vi "WVDIAL_2_Switch_v2.vi"() -> ()   [LabVIEW 2012]
uses:
  <vilib>/DAQmx/create/channels.llb/DAQmx Create Channel (CO-Pulse Generation-Ticks).vi
  <vilib>/DAQmx/configure/timing.llb/DAQmx Timing (Implicit).vi
  <resource>/objmgr/daqmx.rc
  <vilib>/DAQmx/create/channels.llb/DAQmx Create Channel (DO-Digital Output).vi
panel:
  in  "online":u32=2
  in  "offline":u32=2
  out "Error Out":errorcluster
  in  "stop 3":bool
  in  "Error In 3":errorcluster
  out "Error Out 3":errorcluster
  in  "Error In":errorcluster
  in  "Stop":bool
  in  "pulse counter":u32=140 min=4 max=9000 step=1
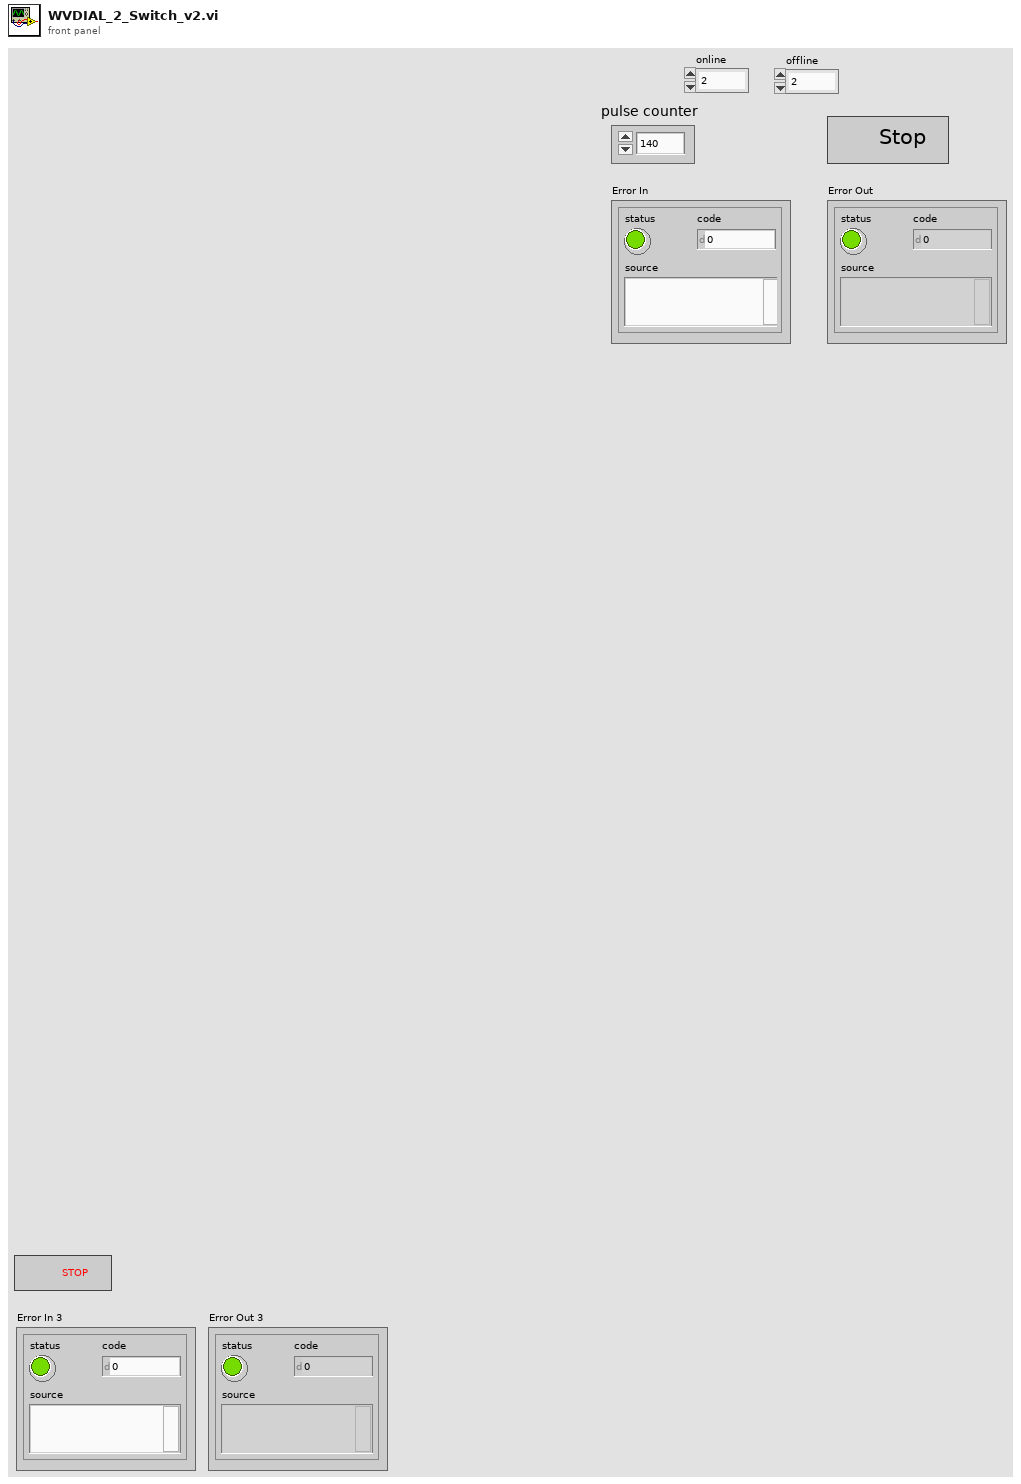
[diagram p1: front panel]
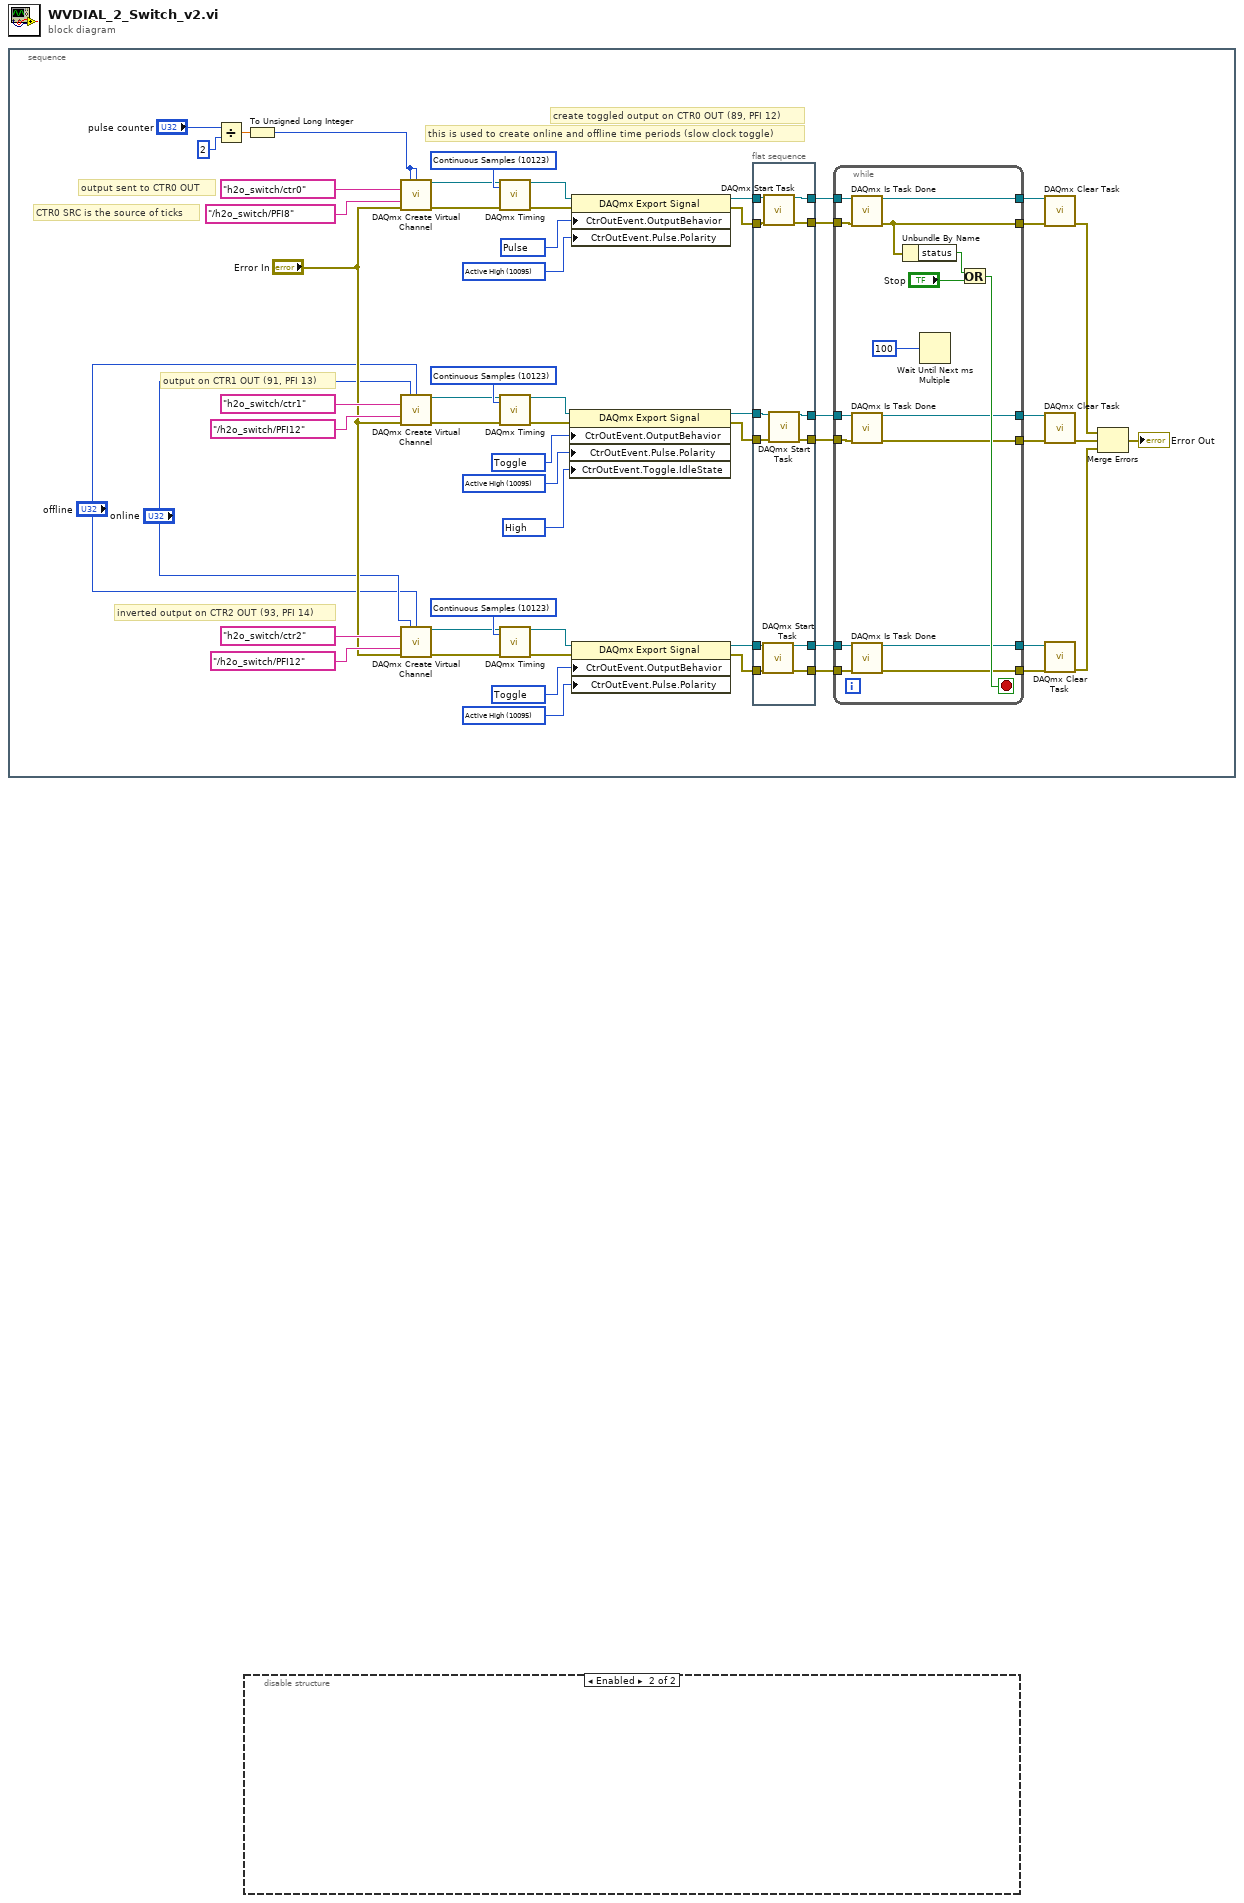
[diagram p0: block diagram]
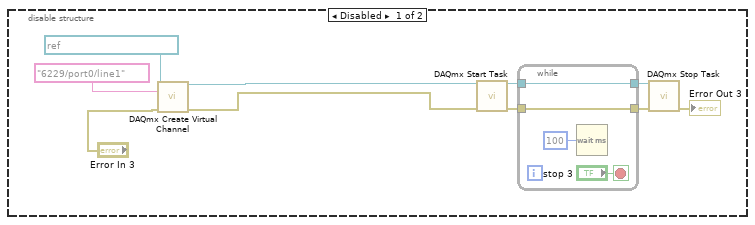
[diagram p2: hidden frame]
diagram:
  n1 = stacked-sequence {
    frame #0 {
      w11 = 10192 items=["High"=10192, "Low"=10214] ("CtrOutEvent.Toggle.IdleState")
      w21 = 10095 items=["Active High"=10095, "Active Low"=10096] ("CtrOutEvent.Pulse.Polarity")
      w27 = 10307 items=["Pulse"=10265, "Toggle"=10307] ("CtrOutEvent.OutputBehavior")
      w24 = 10123 items=["Finite Samples"=10178, "Continuous Samples"=10123, "Hardware Timed Single Point"=12522] ("sample mode")
      w38 = 10095 items=["Active High"=10095, "Active Low"=10096] ("CtrOutEvent.Pulse.Polarity")
      w44 = 10307 items=["Pulse"=10265, "Toggle"=10307] ("CtrOutEvent.OutputBehavior")
      w41 = 10123 items=["Finite Samples"=10178, "Continuous Samples"=10123, "Hardware Timed Single Point"=12522] ("sample mode")
      w45 = 10095 items=["Active High"=10095, "Active Low"=10096] ("CtrOutEvent.Pulse.Polarity")
      w57 = 10265 items=["Pulse"=10265, "Toggle"=10307] ("CtrOutEvent.OutputBehavior")
      w49 = 10123 items=["Finite Samples"=10178, "Continuous Samples"=10123, "Hardware Timed Single Point"=12522] ("sample mode")
      # "inverted output on CTR2 OUT (93, PFI 14)"
      # "output on CTR1 OUT (91, PFI 13)"
      # "output sent to CTR0 OUT"
      # "CTR0 SRC is the source of ticks"
      # "this is used to create online and offline time periods (slow clock toggle)"
      # "create toggled output on CTR0 OUT (89, PFI 12)"
      n2 = Divide(x="pulse counter", y=u32 2) -> (x/y=w9:dbl)
      n3 = To Unsigned Long Integer(number=w9) -> (unsigned 32bit integer=w3:u32)
      n4 = call-poly <vilib>:"DAQmx Create Virtual Channel.vi"("high ticks"=w3, "low ticks"=w3, "counter"=tag "h2o_switch/ctr0", "source of ticks"=tag "/h2o_switch/PFI8", "error in"="Error In") -> ("task out"=w47:refnum<k21>, "error out"=w48:errorcluster)  [unwired: 9 in]
      n5 = call-poly <vilib>:"DAQmx Create Virtual Channel.vi"("high ticks"="online", "low ticks"="offline", "counter"=tag "h2o_switch/ctr1", "source of ticks"=tag "/h2o_switch/PFI12", "error in"="Error In") -> ("task out"=w39:refnum<k21>, "error out"=w40:errorcluster)  [unwired: 9 in]
      n6 = call-poly <vilib>:"DAQmx Create Virtual Channel.vi"("high ticks"="online", "low ticks"="offline", "counter"=tag "h2o_switch/ctr2", "source of ticks"=tag "/h2o_switch/PFI12", "error in"="Error In") -> ("task out"=w22:refnum<k21>, "error out"=w23:errorcluster)  [unwired: 9 in]
      n7 = call-poly <vilib>:"DAQmx Timing.vi"("task/channels in"=w47, "sample mode"=w49, "error in"=w48) -> ("task out"=w55:refnum<k21>, "error out"=w53:errorcluster)  [unwired: 11 in]
      n8 = call-poly <vilib>:"DAQmx Timing.vi"("task/channels in"=w39, "sample mode"=w41, "error in"=w40) -> ("task out"=w43:refnum<k21>, "error out"=w42:errorcluster)  [unwired: 11 in]
      n9 = call-poly <vilib>:"DAQmx Timing.vi"("task/channels in"=w22, "sample mode"=w24, "error in"=w23) -> ("task out"=w26:refnum<k21>, "error out"=w25:errorcluster)  [unwired: 11 in]
      n10 = property class="DAQmx Export Signal"(reference=w43, error in=w42, "CtrOutEvent.OutputBehavior"=w44, "CtrOutEvent.Pulse.Polarity"=w38, "CtrOutEvent.Toggle.IdleState"=w11) -> (reference out=w36:refnum<k21>, error out=w34:errorcluster)
      n11 = property class="DAQmx Export Signal"(reference=w55, error in=w53, "CtrOutEvent.OutputBehavior"=w57, "CtrOutEvent.Pulse.Polarity"=w45) -> (reference out=w56:refnum<k21>, error out=w54:errorcluster)
      n12 = property class="DAQmx Export Signal"(reference=w26, error in=w25, "CtrOutEvent.OutputBehavior"=w27, "CtrOutEvent.Pulse.Polarity"=w21) -> (reference out=w17:refnum<k21>, error out=w16:errorcluster)
      n13 = flat-sequence {
        tunnel: [w67] -> w50
        tunnel: [w66] -> w46
        tunnel: [w64] -> w35
        tunnel: [w62] -> w33
        tunnel: [w59] -> w15
        tunnel: [w58] -> w14
        tunnel: w56 -> [w68]
        tunnel: w54 -> [w69]
        tunnel: w36 -> [w65]
        tunnel: w34 -> [w63]
        tunnel: w17 -> [w61]
        tunnel: w16 -> [w60]
        frame #0 {
          n14 = call <vilib>:"DAQmx Start Task.vi"("task/channels in"=w61, "error in"=w60) -> ("task out"=w59:refnum<k21>, "error out"=w58:errorcluster)  [unwired: 12 in]
          n15 = call <vilib>:"DAQmx Start Task.vi"("task/channels in"=w68, "error in"=w69) -> ("task out"=w67:refnum<k21>, "error out"=w66:errorcluster)  [unwired: 12 in]
          n16 = call <vilib>:"DAQmx Start Task.vi"("task/channels in"=w65, "error in"=w63) -> ("task out"=w64:refnum<k21>, "error out"=w62:errorcluster)  [unwired: 12 in]
        }
      }
      n17 = while {
        tunnel: w50 -> [w85]
        tunnel: w46 -> [w84]
        tunnel: [w81] -> w52
        tunnel: [w82] -> w51
        tunnel: w35 -> [w74]
        tunnel: w33 -> [w75]
        tunnel: [w77] -> w32
        tunnel: [w76] -> w31
        tunnel: w15 -> [w73]
        tunnel: w14 -> [w72]
        tunnel: [w71] -> w13
        tunnel: [w70] -> w12
        stop <- w83 stop-if-true
        n18 = call <vilib>:"DAQmx Is Task Done.vi"("task/channels in"=w85, "error in"=w84) -> ("task out"=w82:refnum<k21>, "error out"=w81:errorcluster)  [unwired: 11 in, 1 out]
        n19 = call <vilib>:"DAQmx Is Task Done.vi"("task/channels in"=w74, "error in"=w75) -> ("task out"=w77:refnum<k21>, "error out"=w76:errorcluster)  [unwired: 11 in, 1 out]
        n20 = call <vilib>:"DAQmx Is Task Done.vi"("task/channels in"=w73, "error in"=w72) -> ("task out"=w71:refnum<k21>, "error out"=w70:errorcluster)  [unwired: 11 in, 1 out]
        n21 = Unbundle By Name(w81) -> ("status"=w80:bool)
        n22 = Wait Until Next ms Multiple(millisecond multiple=u32 100) -> ()  [unwired: 1 out]
        n23 = Or(x=w80, y="Stop") -> (x .or. y?=w83:bool)
      }
      n24 = call <vilib>:"DAQmx Clear Task.vi"("task in"=w51, "error in"=w52) -> ("error out"=w7:errorcluster)  [unwired: 13 in]
      n25 = call <vilib>:"DAQmx Clear Task.vi"("task in"=w32, "error in"=w31) -> ("error out"=w6:errorcluster)  [unwired: 13 in]
      n26 = call <vilib>:"DAQmx Clear Task.vi"("task in"=w13, "error in"=w12) -> ("error out"=w5:errorcluster)  [unwired: 13 in]
      n27 = Merge Errors(w7, w6, w5) -> (→"Error Out":errorcluster)
    }
  }
  n28 = disable-structure shown="Enabled" {
    frame Disabled {
      n29 = call-poly <vilib>:"DAQmx Create Virtual Channel.vi"("task in"=refnum<k21> "MyDigitalOutTask_0", "lines"=tag "6229/port0/line1", "error in"="Error In 3") -> ("task out"=w88:refnum<k21>, "error out"=w87:errorcluster)  [unwired: 11 in]
      n30 = call <vilib>:"DAQmx Start Task.vi"("task/channels in"=w88, "error in"=w87) -> ("task out"=w91:refnum<k21>, "error out"=w92:errorcluster)  [unwired: 12 in]
      n31 = while {
        tunnel: w91 -> [w97]
        tunnel: w92 -> [w96]
        tunnel: [w97] -> w95
        tunnel: [w96] -> w94
        stop <- "stop 3" stop-if-true
        n32 = Wait (ms)(milliseconds to wait=u32 100) -> ()  [unwired: 1 out]
      }
      n33 = call <vilib>:"DAQmx Stop Task.vi"("task/channels in"=w95, "error in"=w94) -> ("error out"=→"Error Out 3":errorcluster)  [unwired: 12 in, 1 out]
    }
    frame Enabled {
    }
  }
